vi "Drive Calibrate.vi"(7 "Description":string, 8 "Command Info In":T2, 10 "reset pods":bool, 11 "Operation":T1=enum."Calibrate") -> (0 "Command Info Out":T2)   [LabVIEW 2020]
doc: "Often used for joystick control, this VI checks to see that the joystick axes are outside the deadband and updates the motors appropriately."
uses:
  <vilib>/Rock Robotics/WPI/Framework/Command Status Info.ctl
  <vilib>/Rock Robotics/WPI/Framework/Completion Status.ctl
  <vilib>/Rock Robotics/WPI/Framework/Completion Notifier.ctl
  Implementation/Drive Operations.ctl
  Implementation/Drive Setpoints.ctl
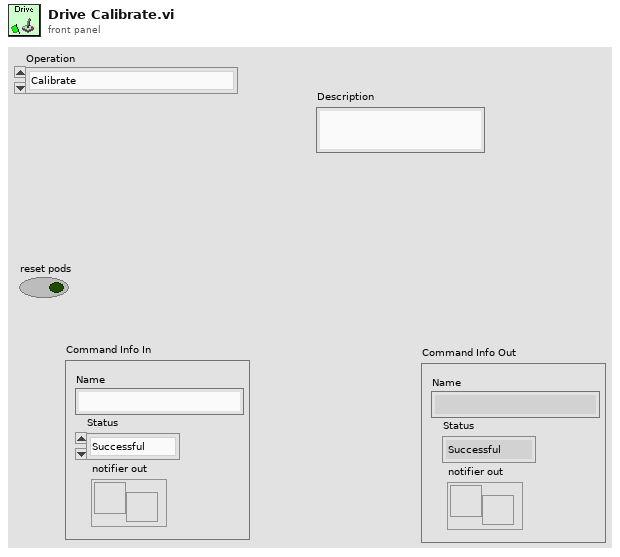
[diagram p1: front panel]
types:
  T1 = typedef "Drive Operations.ctl" = enum16{"Reserve", "Read Current", "Immediate", "Calibrate", "Play Path"}
  T2 = typedef "Command Status Info.ctl" = cluster{"Name":string, "Status":T3, "notifier out":T4}
  T3 = typedef "Completion Status.ctl" = enum16{"Successful", "Aborted", "Incomplete"}
  T4 = typedef "Completion Notifier.ctl" = refnum<notifier>
  T5 = typedef "Drive Setpoints.ctl" = cluster{"Operation":T1, "Trans Vel":cluster{"x":dbl, "y":dbl}, "Rot Vel":cluster{"omega":dbl}, "Swerve Path Data":cluster{"Translations":cluster{"x out":dbl, "y out":dbl}[], "Rotations":cluster{"th":dbl}[]}, "reset pods":bool}
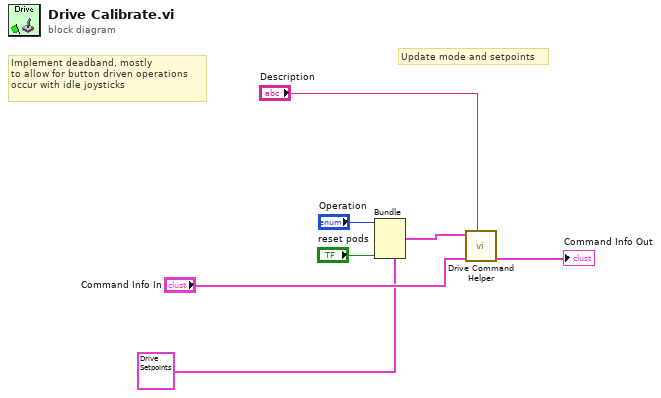
[diagram p0: block diagram]
diagram:
  # "Implement deadband, mostly\nto allow for button driven operations\noccur with idle joysticks"
  # "Update mode and setpoints"
  n1 = Bundle(cluster=T5 {"Operation"=enum."Calibrate", "Trans Vel"={"x"=0.0, "y"=0.0}, "Rot Vel"={"omega"=0.0}, "Swerve Path Data"={"Translations"=[], "Rotations"=[]}, "reset pods"=FALSE} ("SubSystem Data"), "Operation"="Operation", "reset pods"="reset pods") -> (w3:T5)  [unwired: 3 in]
  n2 = call "Drive Command Helper.vi"("Description"="Description", "Command Info In"="Command Info In", "SubSystem Data"=w3) -> ("Command Info Out"=→"Command Info Out":T2)  [unwired: 6 in, 2 out]
